vi "OnTimeoutyes.vi"(0 "CmdLib In":refnum<k24>, 5 "UI":T1, 7 "Status:":refnum<vi>, 9 "In Motion":refnum<vi>, 11 "error in":errorcluster) -> (15 "error out":errorcluster)   [LabVIEW 2021]
uses:
  C:/Program Files/New Focus/New Focus Picomotor Application/Samples/LabVIEW/Model 8742/LabVIEW 2009/CmdLib.dll
  Global Variablesyes.vi
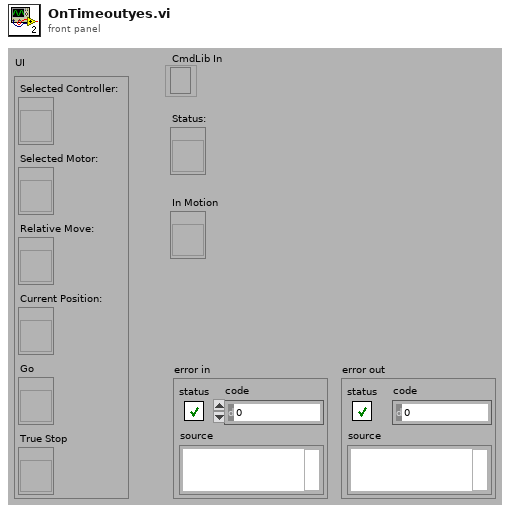
[diagram p1: front panel]
types:
  T1 = cluster{"Selected Controller:":refnum<vi>, "Selected Motor:":refnum<vi>, "Relative Move:":refnum<vi>, "Current Position:":refnum<vi>, "Go":refnum<vi>, "True Stop":refnum<vi>}
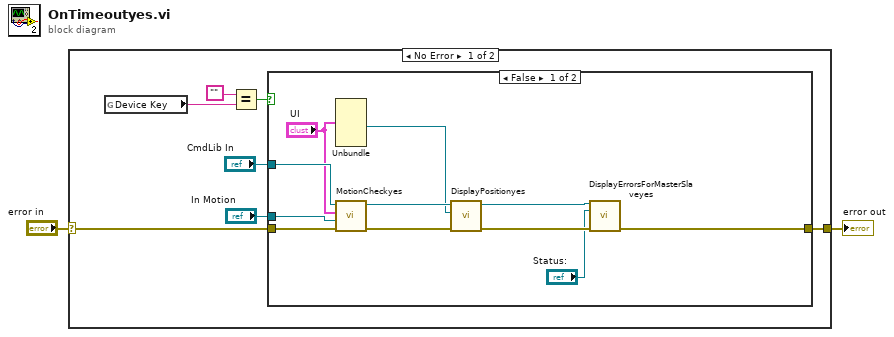
[diagram p0: block diagram]
diagram:
  n1 = case shown="No Error" "error in" {
    selector: "error in" -> [w3 w22]
    tunnel: [w4 w22] -> w2
    frame No Error {
      n2 = global read "Global Variablesyes.vi" "Device Key"() -> (w8:string)
      n3 = Equal?(x="", y=w8) -> (x = y?=w7:bool)
      n4 = case shown="False" w7 {
        tunnel: w3 -> [w19 w21]
        tunnel: [w20 w21] -> w4
        tunnel: "CmdLib In" -> [w16 _]
        tunnel: "In Motion" -> [w13 _]
        frame False {
          n5 = Unbundle("UI") -> ("Current Position:"=w11:refnum<vi>)  [unwired: 5 out]
          n6 = call "MotionCheckyes.vi"("error in (no error)"=w19, "In Motion?"=w13, "UI"="UI", "CmdLib In"=w16) -> ("error out"=w18:errorcluster, "CmdLib Out"=w14:refnum<k24>)  [unwired: 6 in]
          n7 = call "DisplayPositionyes.vi"("error in"=w18, "Current Position:"=w11, "CmdLib In"=w14) -> ("error out"=w17:errorcluster, "CmdLib Out"=w15:refnum<k24>)  [unwired: 7 in]
          n8 = call "DisplayErrorsForMasterSlaveyes.vi"("CmdLib In"=w15, "Status:"="Status:", "error in"=w17) -> ("error out"=w20:errorcluster)  [unwired: 11 in, 1 out]
        }
        frame True {
        }
      }
    }
    frame Error {
    }
  }
  "error out" <- w2
